vi "Diagram Connect Tunnel with Wire.vi"(8 "error in (no error)":errorcluster, 9 "FrontEnd Connected Info":T1[](array[typedef]), 10 "Front Tunnels":refnum<vi>[](array[refnum]), 11 "Diagram in":refnum<vi>) -> (0 "error out":errorcluster, 2 "Array out":i32[](array[numeric]), 3 "Diagram out":refnum<vi>)   [LabVIEW 2020, in "CSM-Helper.lvclass"]
uses:
  CSM-Helper.lvclass
  Typedef/Def-Conncted Information.ctl
  <vilib>/Utility/miscctls.llb/LVPositionTypeDef.ctl
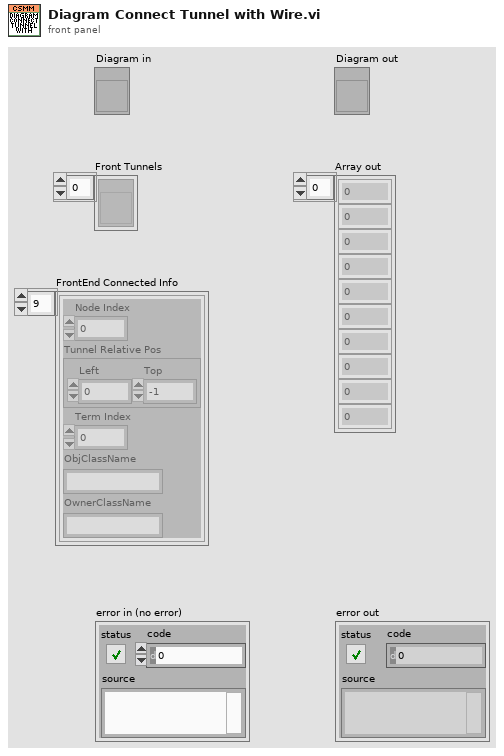
[diagram p1: front panel]
types:
  T1 = typedef "CSM-Helper.lvclass/Def-Conncted Information.ctl" = cluster{"Node Index":i32, "Tunnel Relative Pos":T2, "Term Index":i32, "ObjClassName":string, "OwnerClassName":string}
  T2 = typedef "LVPositionTypeDef.ctl" = cluster{"Left":i32, "Top":i32}
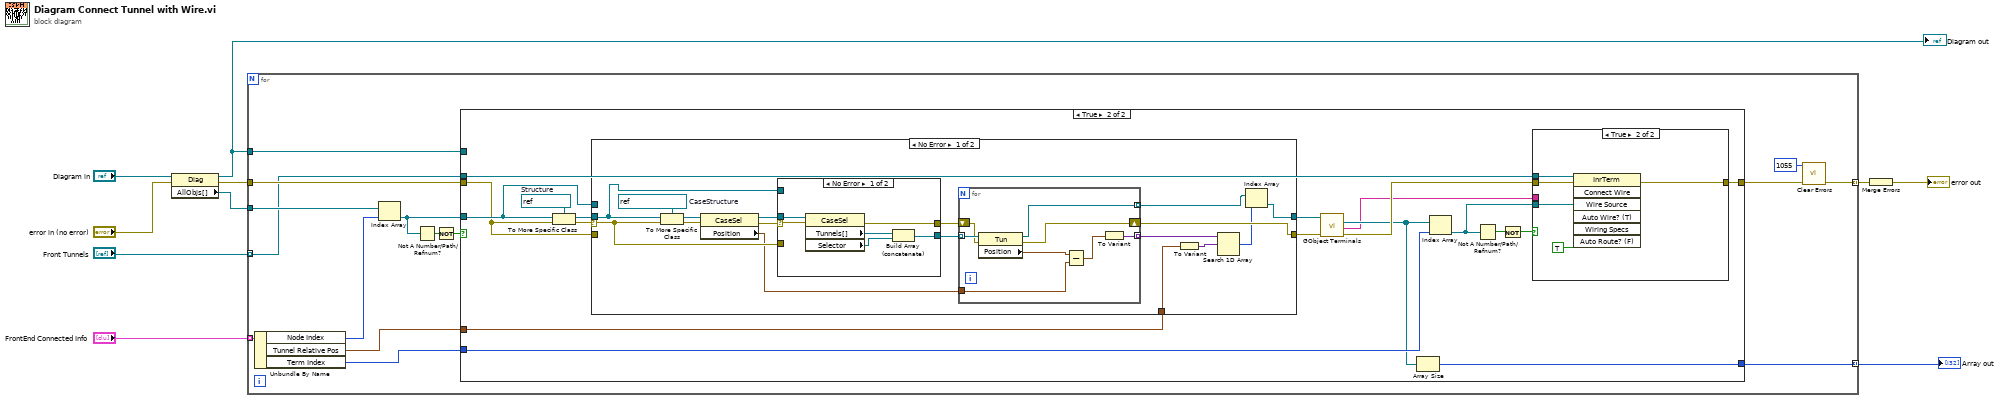
[diagram p0: block diagram]
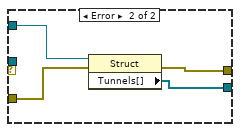
[diagram p3: hidden frame]
diagram:
  n1 = property on="Property Node" class="Diag"(reference="Diagram in", error in="error in (no error)") -> (reference out=w8:refnum<vi>, error out=w10:errorcluster, "AllObjs[]"=w1:refnum<vi>[])
  "Diagram out" <- w8
  n2 = for {
    tunnel: w1 -> [w23]
    tunnel: "FrontEnd Connected Info" -> [w22] mode=indexing
    tunnel: "Front Tunnels" -> [w21] mode=indexing
    tunnel: w10 -> [w25]
    tunnel: [w12] -> w2 mode=indexing
    tunnel: [w18] -> w6 mode=indexing
    tunnel: w8 -> [w17]
    n3 = Unbundle By Name(w22) -> ("Node Index"=w15:i32, "Tunnel Relative Pos"=w13:T2, "Term Index"=w14:i32)
    n4 = Index Array(array=w23, index=w15) -> (element=w19:refnum<vi>)
    n5 = Not A Number/Path/Refnum?(number/path/refnum=w19) -> (NaN/Path/Refnum?=w16:bool)
    n6 = Not(x=w16) -> (.not. x?=w20:bool)
    n7 = case shown="True" w20 {
      tunnel: w25 -> [w26 w28]
      tunnel: [w26 w44] -> w24
      tunnel: w19 -> [_ w29]
      tunnel: w21 -> [_ w42]
      tunnel: [_ w43] -> w18
      tunnel: w17 -> [_ _]
      tunnel: w14 -> [_ w41]
      tunnel: w13 -> [_ w31]
      frame False {
      }
      frame True {
        w34 = refnum<vi> refnum  # Structure
        n8 = To More Specific Class(target class=w34, reference=w29, error in=w28) -> (specific class reference=w35:refnum<vi>, error out=w32:errorcluster)
        n9 = case shown="No Error" w32 {
          selector: w32 -> [w58 _]
          tunnel: w35 -> [w59 _]
          tunnel: [w45 w81] -> w33
          tunnel: w31 -> [w50 _]
          tunnel: [w55 w80] -> w30
          tunnel: w29 -> [_ w81]
          tunnel: w28 -> [_ w80]
          frame No Error {
            w60 = refnum<vi> refnum  # CaseStructure
            n10 = To More Specific Class(target class=w60, reference=w59, error in=w58) -> (specific class reference=w61:refnum<vi>, error out=w53:errorcluster)
            n11 = property class="CaseSel"(reference=w61, error in=w53) -> (reference out=w54:refnum<vi>, error out=w52:errorcluster, "Position"=w51:T2)
            n12 = case shown="No Error" w52 {
              selector: w52 -> [w73 _]
              tunnel: [w74 w79] -> w56
              tunnel: w54 -> [w72 _]
              tunnel: [w71 w76] -> w57
              tunnel: w59 -> [_ w78]
              tunnel: w58 -> [_ w77]
              frame No Error {
                n13 = property class="CaseSel"(reference=w72, error in=w73) -> (error out=w74:errorcluster, "Tunnels[]"=w75:refnum<vi>[], "Selector"=w70:refnum<vi>)  [unwired: 1 out]
                n14 = Build Array (concatenate)(w75, w70) -> (w71:refnum<vi>[])
              }
              frame Error {
                n15 = property class="Struct"(reference=w78, error in=w77) -> (error out=w79:errorcluster, "Tunnels[]"=w76:refnum<vi>[])  [unwired: 1 out]
              }
            }
            n16 = for {
              tunnel: w57 -> [w69] mode=indexing
              tunnel: [w63] -> w49 mode=indexing
              shift-right: [w67] -> w55
              shift-left: w56 -> [w68]
              tunnel: w51 -> [w65]
              tunnel: [w62] -> w47 mode=indexing
              n17 = property class="Tun"(reference=w69, error in=w68) -> (reference out=w62:refnum<vi>, error out=w67:errorcluster, "Position"=w66:T2)
              n18 = Subtract(x=w66, y=w65) -> (x-y=w64:T2)
              n19 = To Variant(anything=w64) -> (Variant=w63:variant)
            }
            n20 = To Variant(anything=w50) -> (Variant=w48:variant)
            n21 = Search 1D Array(1D array=w49, element=w48) -> (index of element=w46:i32)  [unwired: 1 in]
            n22 = Index Array(array=w47, index=w46) -> (element=w45:refnum<vi>)
          }
          frame Error {
          }
        }
        n23 = call "GObject Terminals.vi"("error in (no error)"=w30, "GObject in"=w33) -> ("error in (no error) (dup)"=w37:errorcluster, "Class Name"=w27:string, "Terms[]"=w36:refnum<vi>[])  [unwired: 5 in, 2 out]
        n24 = Array Size(array=w36) -> (size(s)=w43:i32)
        n25 = Index Array(array=w36, index=w41) -> (element=w38:refnum<vi>)
        n26 = Not A Number/Path/Refnum?(number/path/refnum=w38) -> (NaN/Path/Refnum?=w40:bool)
        n27 = Not(x=w40) -> (.not. x?=w39:bool)
        n28 = case shown="True" w39 {
          tunnel: w37 -> [w82 w87]
          tunnel: [w82 w83] -> w44
          tunnel: w42 -> [_ w85]
          tunnel: w38 -> [_ w84]
          tunnel: w27 -> [_ _]
          frame False {
          }
          frame True {
            n29 = invoke class="InrTerm" method="Connect Wire"(reference=w85, error in=w87, "Wire Source"=w84, "Auto Route? (F)"=TRUE) -> (error out=w83:errorcluster)  [unwired: 3 in, 6 out]
          }
        }
      }
    }
    n30 = call <vilib>:"Clear Errors.vi"("error in (no error)"=w24, "specific error code to clear (0: all)"=1055) -> ("error out"=w12:errorcluster)  [unwired: 4 in, 1 out]
  }
  "Array out" <- w6
  n31 = Merge Errors(w2) -> (→"error out":errorcluster)
